vi "PE7265_Check_Queue.vi"(7 "error in (no error)":errorcluster, 10 "queue":refnum<queue>) -> (0 "error out":errorcluster, 2 "PE7265-Cluster":T1={"Lockin 1"=[], "X1-Display"=0.0, "X1 Percent"=0.0, "Y1-Display"=0.0, "X1 Percent 2"=0.0, "Unit X1"="nV", "Unit X1a"="nV", "Unit X2"="nV", "Unit X2a"="nV", "X1 Overload"=FALSE, "Y1 Overload"=FALSE, "Sensitivity Setpoint"=26, "X1"=0.0, "Y1"=0.0} {"Sensitivity Setpoint" items=["2 nV", "5 nV", "10 nV", "20 nV", "50 nV", "100 nV", "200 nV", "500 nV", "1 µV", "2 µV", "5 µV", "10 µV", "20 µV", "50 µV", "100 µV", "200 µV", "500 µV", "1 mV", "2 mV", "5 mV", "10 mV", "20 mV", "50 mV", "100 mV", "200 mV", "500 mV", "1 V", ""]; "X1 Percent 2" scale=0.0..1.0; "X1 Percent" scale=0.0..1.0; "X1-Display" format="%#4_5f"}, 3 "New Entries?":bool)   [LabVIEW 2018]
uses:
  PE7265/PE7265-Cluster.ctl
panel:
  out "Numeric":i32
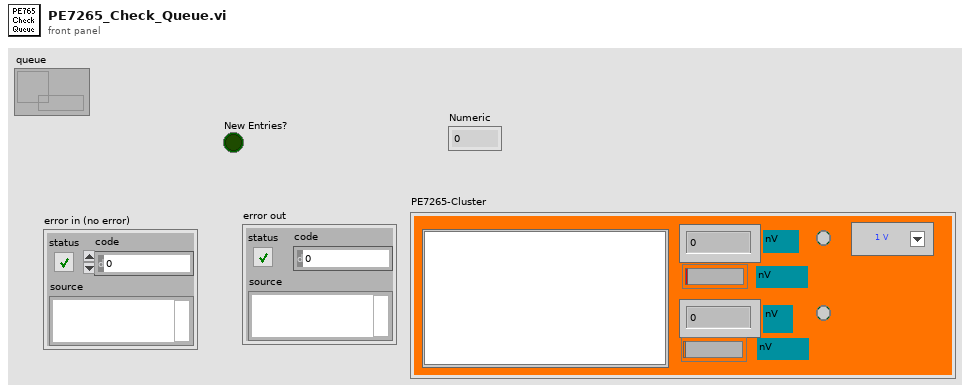
[diagram p1: front panel]
types:
  T1 = typedef "PE7265-Cluster.ctl" = cluster{"Lockin 1":dbl[][], "X1-Display":dbl, "X1 Percent":dbl, "Y1-Display":dbl, "X1 Percent 2":dbl, "Unit X1":string, "Unit X1a":string, "Unit X2":string, "Unit X2a":string, "X1 Overload":bool, "Y1 Overload":bool, "Sensitivity Setpoint":i16, "X1":dbl, "Y1":dbl}
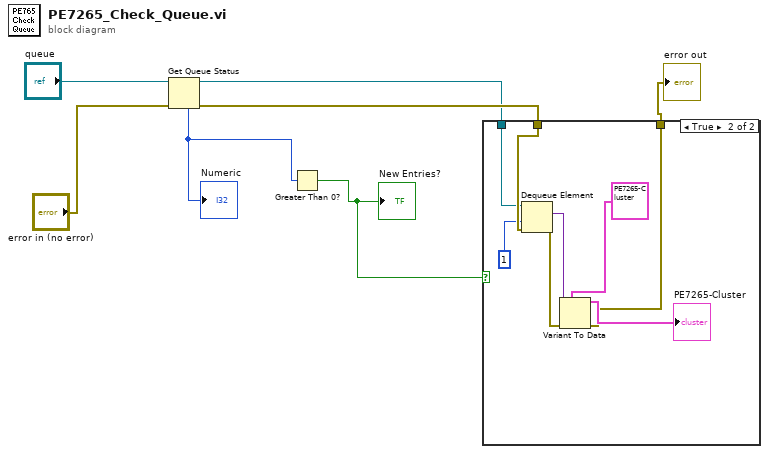
[diagram p0: block diagram]
diagram:
  n1 = Get Queue Status(queue="queue", error in (no error)="error in (no error)") -> (queue out=w1:refnum<queue>, error out=w3:errorcluster, # elements in queue=w5:i32)  [unwired: 1 in, 5 out]
  "Numeric" <- w5
  n2 = Greater Than 0?(x=w5) -> (x > 0?=w4:bool)
  "New Entries?" <- w4
  n3 = case shown="True" w4 {
    tunnel: w3 -> [w8 w14]
    tunnel: [w8 w12] -> w2
    tunnel: w1 -> [_ w11]
    frame False {
    }
    frame True {
      n4 = Dequeue Element(queue=w11, timeout in ms (-1)=1, error in (no error)=w14) -> (element=w10:variant, error out=w13:errorcluster)  [unwired: 2 out]
      n5 = Variant To Data(error in=w13, type=T1 {"Lockin 1"=[], "X1-Display"=0.0, "X1 Percent"=0.0, "Y1-Display"=0.0, "X1 Percent 2"=0.0, "Unit X1"="nV", "Unit X1a"="nV", "Unit X2"="nV", "Unit X2a"="nV", "X1 Overload"=FALSE, "Y1 Overload"=FALSE, "Sensitivity Setpoint"=26, "X1"=0.0, "Y1"=0.0} ("PE7265-Cluster"), Variant=w10) -> (data=→"PE7265-Cluster":T1, error out=w12:errorcluster)
    }
  }
  "error out" <- w2
